vi "EndpointRead.vi"(6 "abort (F)":bool, 7 "timeout in ms (-1)":i32=-1, 11 "channel in":T1) -> (0 "missed":i32, 1 "element out":T2, 4 "aborted?":bool, 5 "timedout?":bool)   [LabVIEW 2020, in "Flex.lvlib"]
uses:
  Flex.lvlib
  ChannelOp.ctl
  <resource>/ChannelSupport/_ChannelSupport/_ChannelSupport.lvlib
  Element.ctl
  ))Channel.ctl
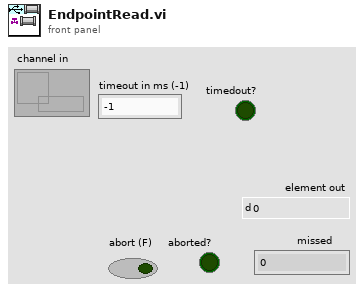
[diagram p1: front panel]
types:
  T1 = typedef "Flex.lvlib/))Channel.ctl" = refnum<queue>
  T2 = typedef "Flex.lvlib/Element.ctl" = dbl
  T3 = typedef "Flex.lvlib/ChannelOp.ctl" = enum16{"Init", "Publish", "Latest", "Next", "Close", "Probe"}
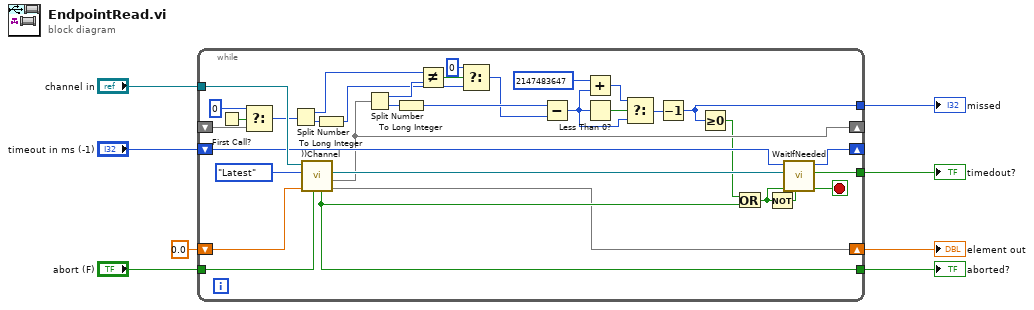
[diagram p0: block diagram]
diagram:
  n1 = while {
    tunnel: [w30] -> w8
    tunnel: "channel in" -> [w42]
    shift-right: [w38] -> _
    shift-left: "timeout in ms (-1)" -> [w39]
    tunnel: [w34] -> w3
    tunnel: "abort (F)" -> [w40]
    tunnel: [w36] -> w5
    shift-right: [w32] -> _
    shift-left: _ -> [w12]
    shift-right: [w33] -> w2
    shift-left: T2 0.0 ("element out") -> [w9]
    stop <- w35 stop-if-true
    n2 = First Call?() -> (First Call?: T/F=w13:bool)
    n3 = Select(t=u64 0, s=w13, f=w12) -> (s? t:f=w11:u64)
    n4 = Split Number(x=w11) -> (hi(x)=w18:u32, lo(x)=w22:u32)
    n5 = call "))Channel.vi"("abort (F)"=w40, "element in"=w9, "channelOp"=ChannelOp."Latest", "channel in"=w42) -> (0:w33, 1:w32, "wait"=w37:refnum<k4>, "aborted?"=w36:bool)  [unwired: 2 in, 2 out]
    n6 = To Long Integer(number=w22) -> (32bit integer=w16:i32)
    n7 = Split Number(x=w32) -> (hi(x)=w19:u16, lo(x)=w21:u16)
    n8 = To Long Integer(number=w21) -> (32bit integer=w20:i32)
    n9 = Not Equal?(x=w18, y=w19) -> (x != y?=w17:bool)
    n10 = Select(t=0, s=w17, f=w16) -> (s? t:f=w15:i32)
    n11 = Subtract(x=w20, y=w15) -> (x-y=w27:i32)
    n12 = Add(x=2147483647, y=w27) -> (x+y=w26:i32)
    n13 = Less Than 0?(x=w27) -> (x < 0?=w29:bool)
    n14 = Select(t=w26, s=w29, f=w27) -> (s? t:f=w28:i32)
    n15 = Decrement(x=w28) -> (x-1=w30:i32)
    n16 = Greater Or Equal To 0?(x=w30) -> (x >= 0?=w31:bool)
    n17 = Or(x=w31, y=w36) -> (x .or. y?=w24:bool)
    n18 = Not(x=w24) -> (.not. x?=w23:bool)
    n19 = call <resource>:"WaitIfNeeded.vi"("retry"=w23, "stopping"=w24, "wait"=w37, "_timeout (ms) in"=w39) -> ("stop loop"=w35:bool, "timed out"=w34:bool, "_timeout (ms) out"=w38:i32)  [unwired: 5 in]
  }
  "element out" <- w2
  "missed" <- w8
  "timedout?" <- w3
  "aborted?" <- w5
